vi "lp-server-events.vi"() -> ()   [LabVIEW 2014]
uses:
  lvnanomsg/socket_options.ctl
  lvnanomsg/nanomsg_context.lvclass
  lvnanomsg/nanomsg_socket.lvclass
  lvnanomsg/nanomsg.lvlib
panel:
  out "element":string
  out "time (ms)":u32
  in  "stop?":bool
  in  "endpoint":string="tcp://127.0.0.1:5555"
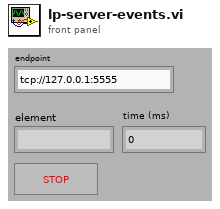
[diagram p1: front panel]
types:
  T1 = typedef "nanomsg.lvlib/socket_options.ctl" = u16
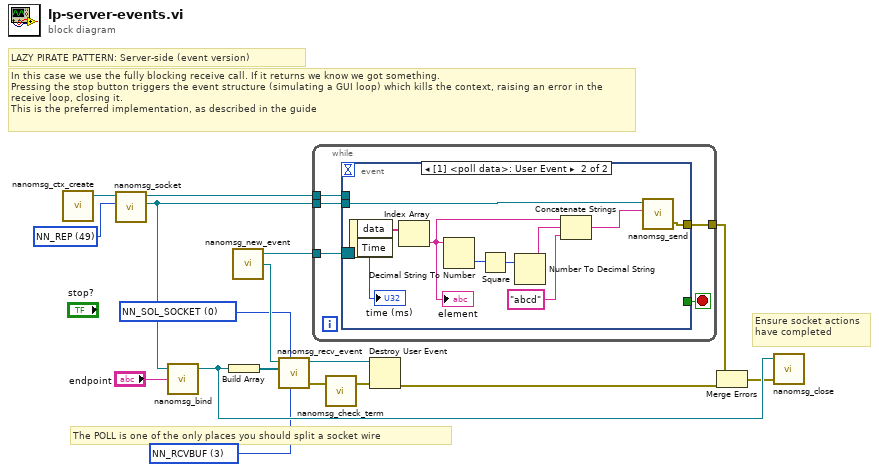
[diagram p0: block diagram]
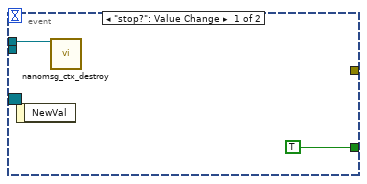
[diagram p2: hidden frame]
diagram:
  w1 = T1 3 items=["NN_LINGER"=1, "NN_SNDBUF"=2, "NN_RCVBUF"=3, "NN_SNDTIMEO"=4, "NN_RCVTIMEO"=5, "NN_RECONNECT_IVL"=6, "NN_RECONNECT_IVL_MAX"=7, "NN_SNDPRIO"=8, "NN_RCVPRIO"=9, "NN_SNDFD"=10, "NN_RCVFD"=11, "NN_DOMAIN"=12, "NN_PROTOCOL"=13, "NN_IPV4ONLY"=14, "NN_SOCKET_NAME"=15, "NN_RCVMAXSIZE"=16, "NN_MAXTTL"=17] ("Socket option")
  w2 = 0 items=["NN_WS"=-4, "NN_TCP"=-3, "NN_IPC"=-2, "NN_INPROC"=-1, "NN_SOL_SOCKET"=0, "NN_PAIR"=16, "NN_PUB"=32, "NN_SUB"=33, "NN_REQ"=48, "NN_REP"=49, "NN_PUSH"=80, "NN_PULL"=81, "NN_SURVEYOR"=98, "NN_RESPONDENT"=99, "NN_BUS"=112] ("socket levels")
  w3 = 49 items=["NN_WS"=-4, "NN_TCP"=-3, "NN_IPC"=-2, "NN_INPROC"=-1, "NN_SOL_SOCKET"=0, "NN_PAIR"=16, "NN_PUB"=32, "NN_SUB"=33, "NN_REQ"=48, "NN_REP"=49, "NN_PUSH"=80, "NN_PULL"=81, "NN_SURVEYOR"=98, "NN_RESPONDENT"=99, "NN_BUS"=112] ("socket type")
  # "Ensure socket actions have completed"
  # "The POLL is one of the only places you should split a socket wire"
  # "In this case we use the fully blocking receive call. If it returns we know we got something.\nPressing the stop button triggers the event structure (simulating a GUI loop) which kills the context, raising an error in the receive loop, closing it.\nThis is the preferred implementation, as described in the guide"
  # "LAZY PIRATE PATTERN: Server-side (event version)"
  n1 = call "nanomsg_ctx_create.vi"() -> ("context out"=w16:refnum<class "nanomsg_context.lvclass">)  [unwired: 4 in, 1 out]
  n2 = call "nanomsg_socket.vi"("socket type"=w3, "context in"=w16) -> ("socket out"=w11:refnum<class "nanomsg_socket.lvclass">, "context out"=w15:refnum<class "nanomsg_context.lvclass">)  [unwired: 3 in, 1 out]
  n3 = call "nanomsg_bind.vi"("endpoint"="endpoint", "socket in"=w11) -> ("socket out"=w10:refnum<class "nanomsg_socket.lvclass">)  [unwired: 2 in, 1 out]
  n4 = Build Array(w10) -> (w14:refnum<class "nanomsg_socket.lvclass">[])
  n5 = call "nanomsg_new_event.vi"() -> ("user event"=w12:refnum<user-event>, "event ref out"=w13:refnum<event-registration>)  [unwired: 3 in, 1 out]
  n6 = call "nanomsg_recv_event.vi"("options"=w1, "level"=w2, "sockets"=w14, "poll event"=w12) -> ("error out"=w9:errorcluster, "poll event out"=w8:refnum<user-event>)  [unwired: 3 in, 1 out]
  n7 = while {
    tunnel: w15 -> [w22]
    tunnel: w13 -> [w21]
    tunnel: w11 -> [w20]
    tunnel: [w18] -> w6
    stop <- w19 stop-if-true
    n8 = event shown="[1] <poll data>: User Event" {
      selector: w21 -> [_ _]
      dyn-events: _ -> [_ _]
      timeout: _ -> [_ _]
      tunnel: w22 -> [w24 _]
      tunnel: w20 -> [_ w29]
      tunnel: [TRUE ("NewVal") _] -> w19
      tunnel: [_ w27] -> w18
      event "stop?": Value Change {
        n9 = event-data() -> ()  [unwired: 1 in, 1 out]
        n10 = call "nanomsg_ctx_destroy.vi"("context in"=w24) -> ()  [unwired: 4 in, 1 out]
      }
      event User Event {
        n11 = event-data() -> ("data"=w31:string[], "Time"=→"time (ms)":u32)  [unwired: 1 in]
        n12 = Index Array(array=w31) -> (element=w30:string)  [unwired: 1 in]
        "element" <- w30
        n13 = Decimal String To Number(string=w30) -> (number=w32:i32)  [unwired: 2 in, 1 out]
        n14 = Square(x=w32) -> (x^2=w33:i32)
        n15 = Number To Decimal String(number=w33) -> (decimal integer string=w34:string)  [unwired: 1 in]
        n16 = Concatenate Strings(w30, w34, "abcd") -> (w25:string)
        n17 = call "nanomsg_send.vi"("data"=w25, "socket in"=w29) -> ("error out"=w27:errorcluster)  [unwired: 2 in, 1 out]
      }
    }
  }
  n18 = call "nanomsg_check_term.vi"("error in"=w9) -> ("error out"=w7:errorcluster)  [unwired: 1 in, 1 out]
  n19 = Destroy User Event(user event=w8, error in=w7) -> (error out=w5:errorcluster)
  n20 = Merge Errors(w6, w5) -> (w4:errorcluster)
  n21 = call "nanomsg_close.vi"("error in"=w4, "socket"=w10) -> ()  [unwired: 3 in, 1 out]
